vi "Get By ID.vi"(8 "error in (no error)":errorcluster, 10 "ID":i64, 11 "Submission DB in":refnum<class "Submission DB.lvclass">) -> (0 "error out":errorcluster, 2 "Submission":refnum<class "Submission.lvclass">, 3 "Submission DB out":refnum<class "Submission DB.lvclass">)   [LabVIEW 2020, in "Summer of LabVIEW.lvlib" / "Submission DB.lvclass"]
uses:
  Submission DB.lvclass
  Submission DB.lvclass/Submission DB.ctl
  Submission/Submission.lvclass
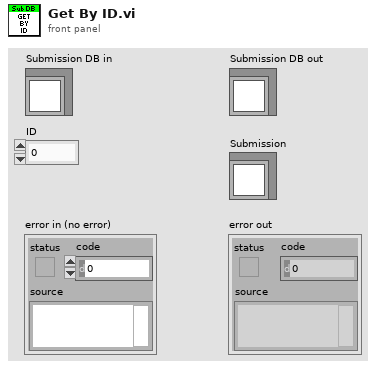
[diagram p1: front panel]
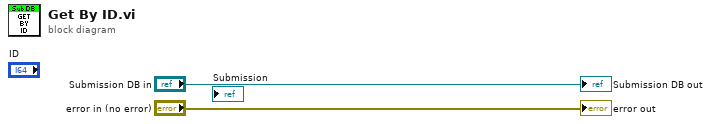
[diagram p0: block diagram]
diagram:
  "error out" <- "error in (no error)"
  "Submission DB out" <- "Submission DB in"
